vi "test caller.vi"() -> ()   [LabVIEW 2020]
uses:
  <userlib>/_NEVSTOP/Communicable State Machine(CSM)/Communicable State Machine.lvlib
  <userlib>/_NEVSTOP/Communicable State Machine(CSM)/_csmHelper/CSM-Helper.lvclass
  <userlib>/_NEVSTOP/Communicable State Machine(CSM)/_csmHelper/API/Destroy.vi
  <userlib>/_NEVSTOP/Communicable State Machine(CSM)/_csmHelper/API/Create From VI Reference.vi
  <userlib>/_NEVSTOP/Communicable State Machine(CSM)/_csmHelper/Properties/Read Back Tunnels Refs.vi
  <userlib>/_NEVSTOP/Communicable State Machine(CSM)/_Polymophic/Build No-Reply Asynchronous Message with Arguments.vi
panel:
  out "Array":string[](array[string])
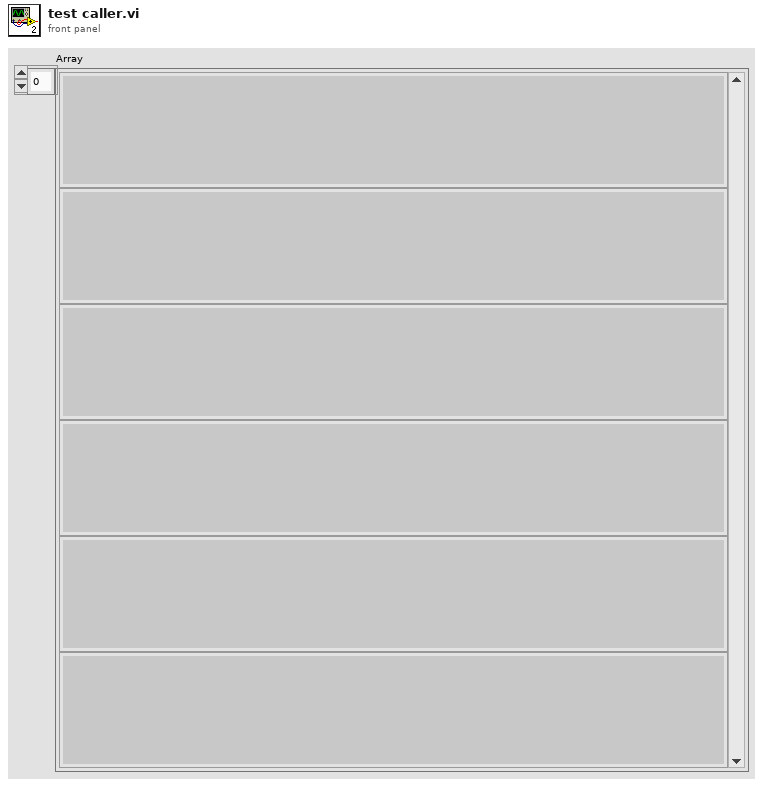
[diagram p1: front panel]
types:
  T1 = enum32{"Invalid", "Standard", "Closed", "Hidden", "Minimized", "Maximized"}
  T2 = enum32{"invalid app kind", "Development System", "Run Time System", "Student Edition", "Embedded LabVIEW", "Evaluation", "Custom"}
  T3 = typedef "Communicable State Machine.lvlib/_CSM_Response Source Message.ctl" = cluster{"‘State":string, "’Arguments":string, "’Error":errorcluster}
  T4 = cluster{"Core":cluster{"Current VI Reference":refnum<vi>, "Close Panel on Exit?":bool}, "Your Boolean data":bool, "Your string data":string}
  T5 = cluster{"Current VI Reference":refnum<vi>, "Close Panel on Exit?":bool}
  T6 = typedef "CSM-Helper.lvclass/_csmhelper_Back_Tunnels_Refs.ctl" = cluster{"Registration":refnum<vi>, "InternalData":refnum<vi>, "Resp":refnum<vi>, "Remaining State":refnum<vi>, "Error":refnum<vi>}
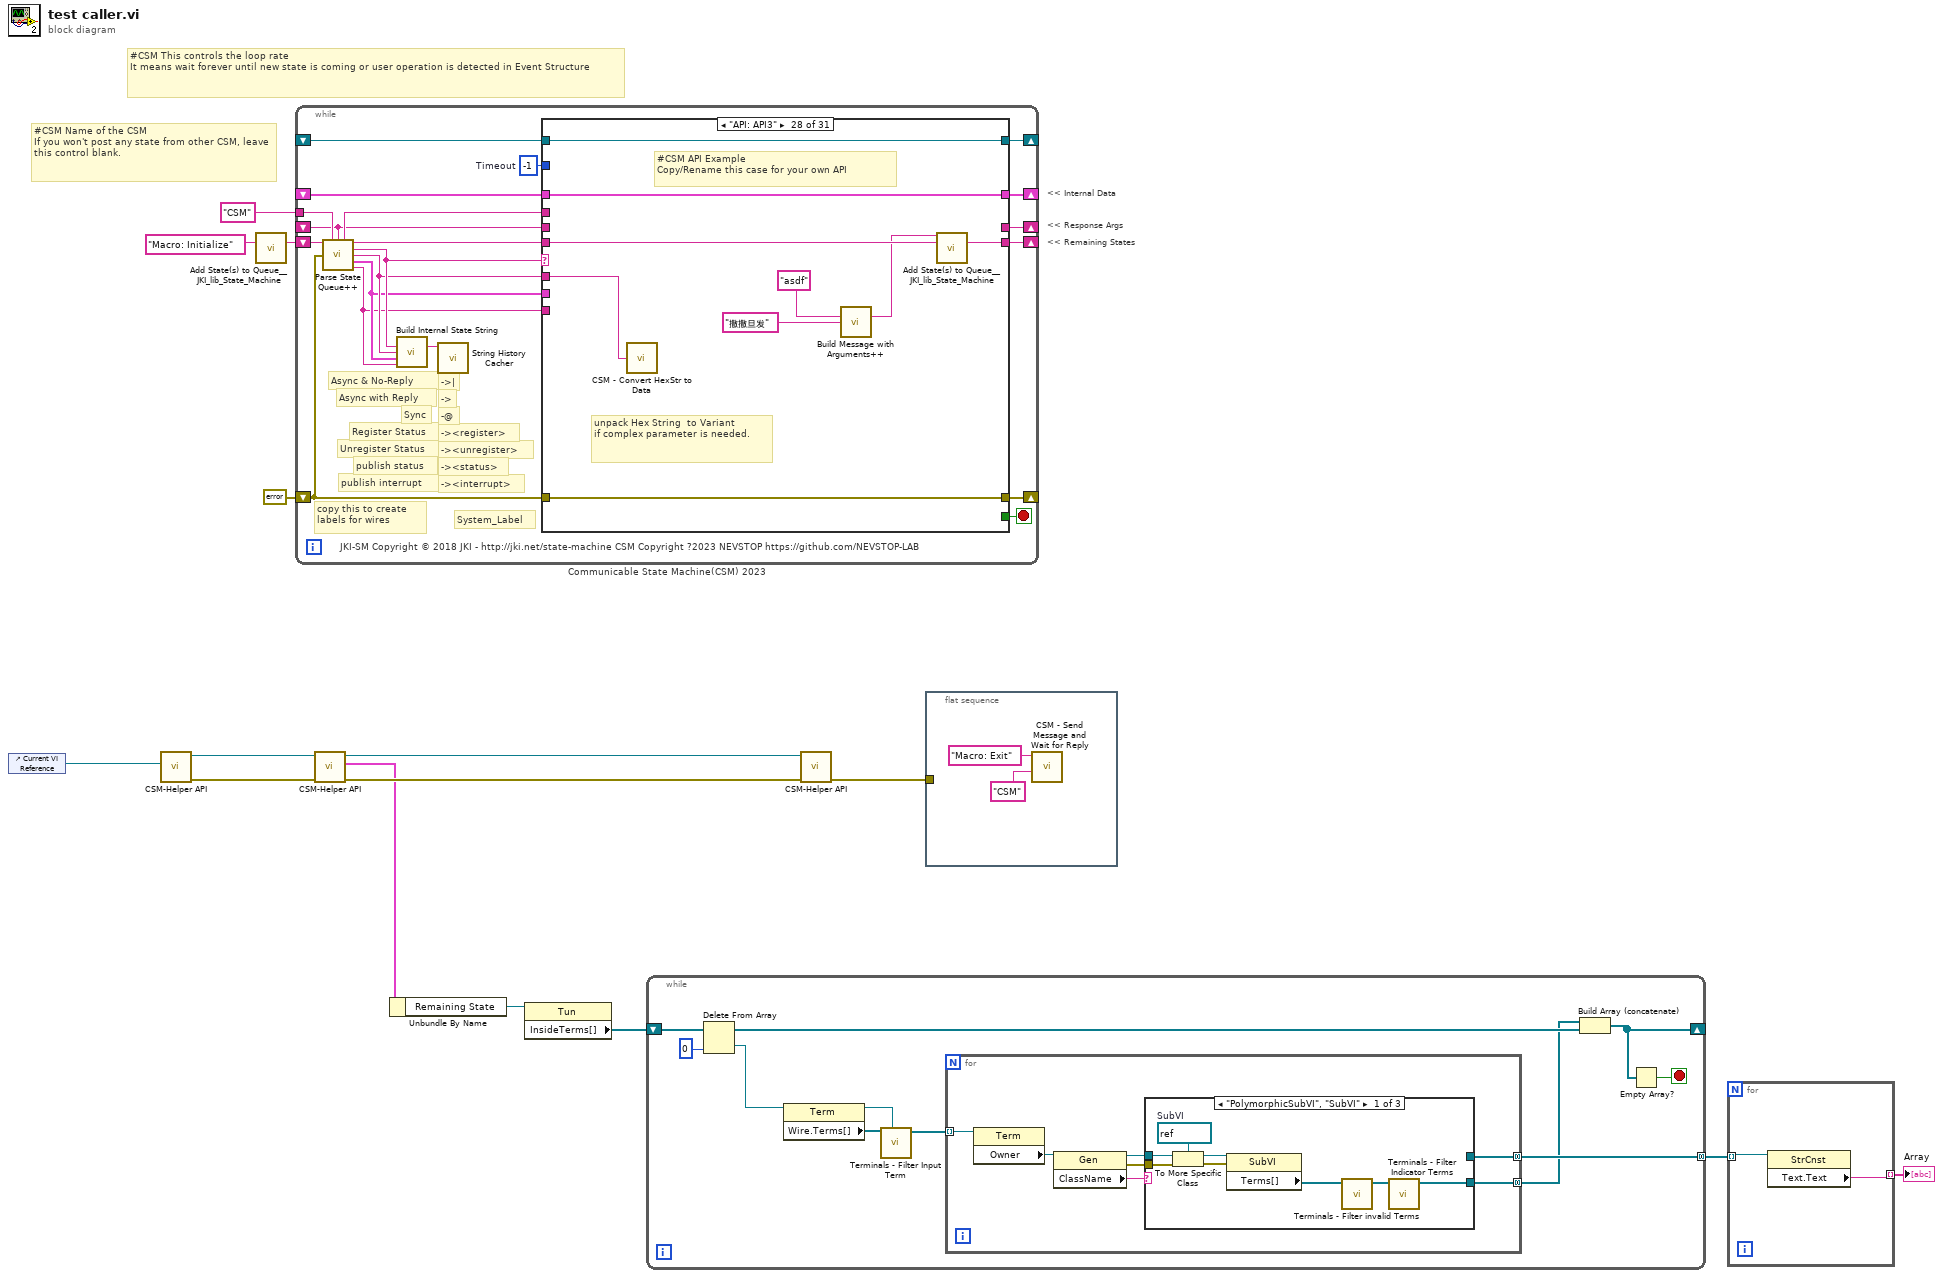
[diagram p0: block diagram]
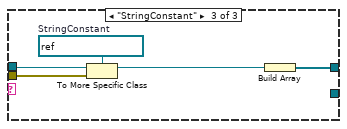
[diagram p3: hidden frame]
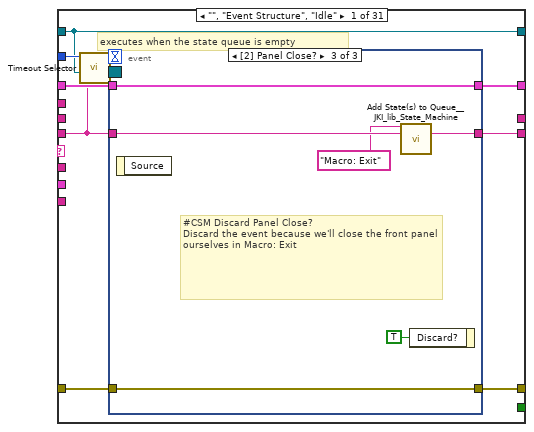
[diagram p4: hidden frame]
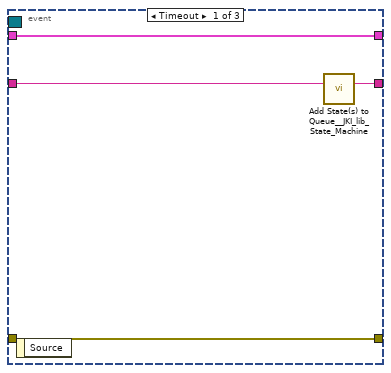
[diagram p5: hidden frame]
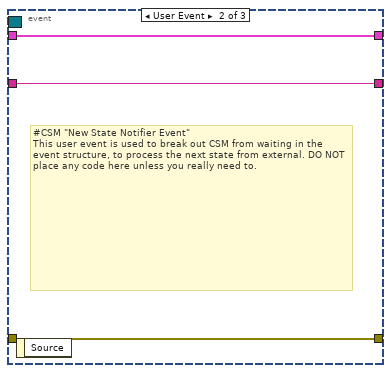
[diagram p6: hidden frame]
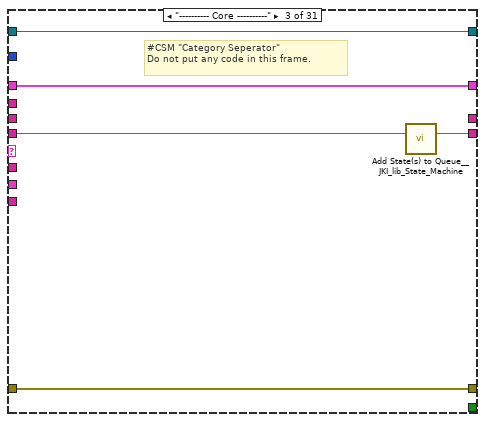
[diagram p8: hidden frame]
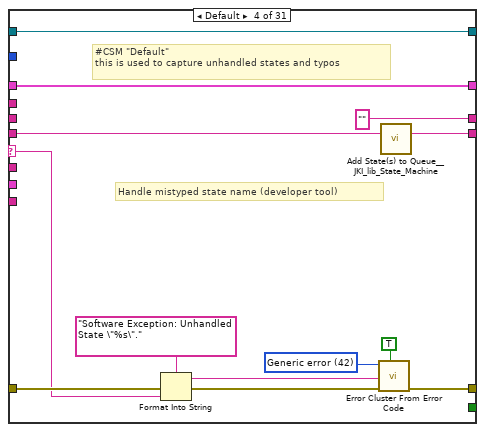
[diagram p9: hidden frame]
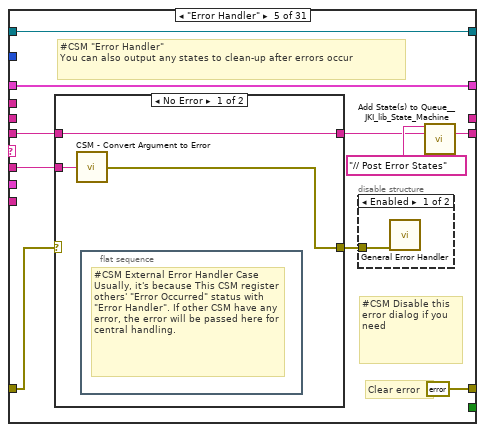
[diagram p10: hidden frame]
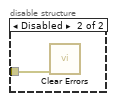
[diagram p11: hidden frame]
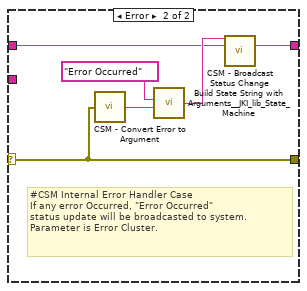
[diagram p12: hidden frame]
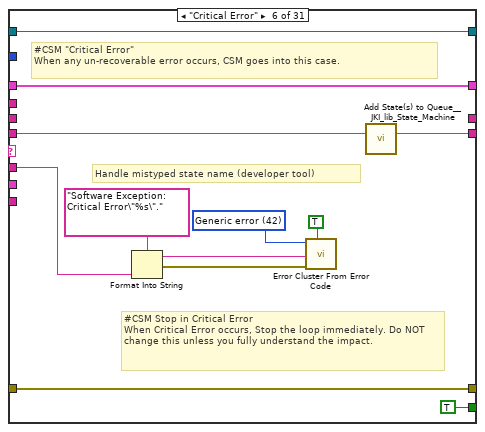
[diagram p13: hidden frame]
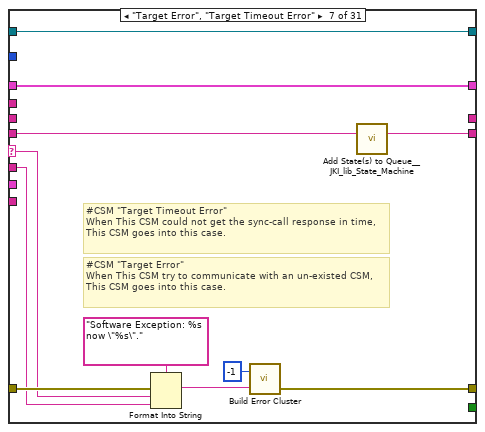
[diagram p14: hidden frame]
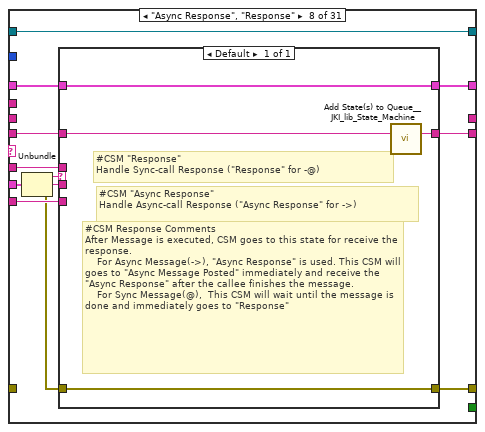
[diagram p15: hidden frame]
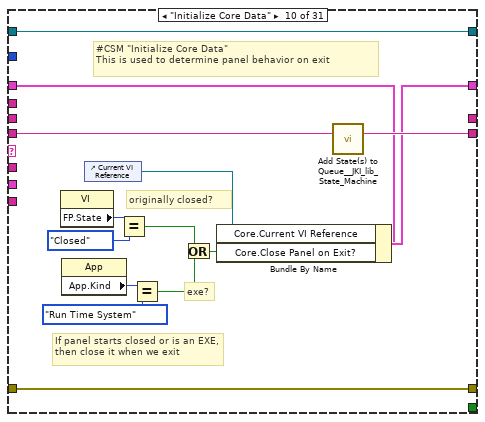
[diagram p17: hidden frame]
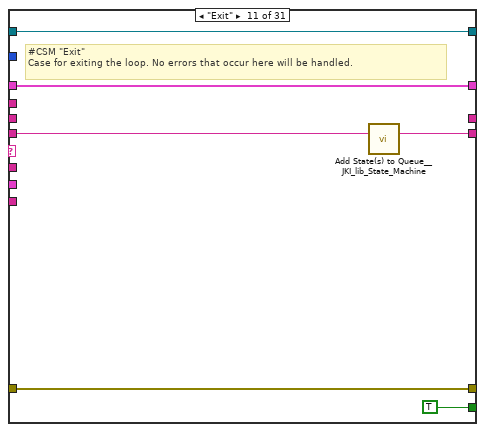
[diagram p18: hidden frame]
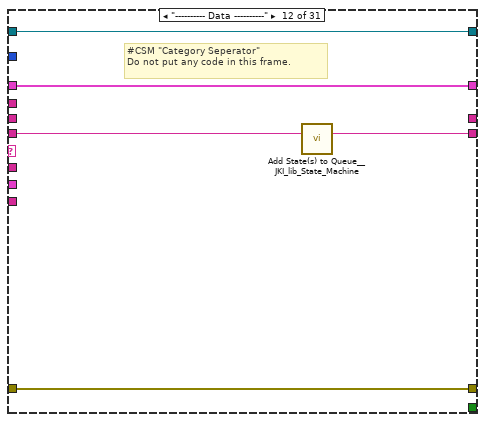
[diagram p19: hidden frame]
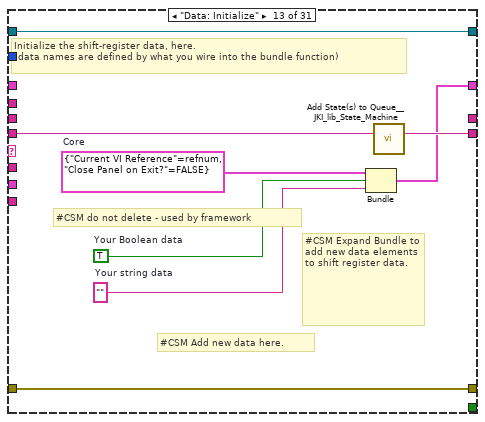
[diagram p20: hidden frame]
diagram:
  # "#CSM Name of the CSM\nIf you won't post any state from other CSM, leave this control blank."
  # "#CSM This controls the loop rate\nIt means wait forever until new state is coming or user operation is detected in Event Structure"
  # "<< Internal Data"
  # "<< Response Args"
  # "<< Remaining States"
  n1 = control-ref of="Current VI Reference"() -> (w15:refnum<vi>)
  n2 = call-poly <userlib>:"CSM-Helper API.vi"("VI"=w15) -> ("error out"=w9:errorcluster, "CSM-Helper.lvclass"=w8:refnum<class "CSM-Helper.lvclass">)  [unwired: 9 in]
  n3 = call <vilib>:"Add State(s) to Queue__JKI_lib_State_Machine.vi"("State(s) in (\"\")"="Macro: Initialize" ("Init State(\"Macro: Initialize\")")) -> ("States Out"=w10:string)  [unwired: 14 in]
  n4 = while "Communicable State Machine(CSM) 2023" {
    shift-right: [w30] -> _
    shift-left: _ -> [w29]
    shift-right: [w33] -> _
    shift-left: errorcluster {"status"=FALSE, "code"=0, "source"=""} ("error out") -> [w27]
    shift-right: [w32] -> _
    shift-left: w10 -> [w34]
    tunnel: "CSM" ("Name(\"\" to use uuid)") -> [w23]
    shift-right: [w26] -> _
    shift-left: _ -> [w16]
    shift-right: [w25] -> _
    shift-left: _ -> [w24]
    stop <- w31 stop-if-true
    w28 = -1  # Timeout
    # "-><interrupt>"
    # "-><status>"
    # "-><unregister>"
    # "-><register>"
    # "-@"
    # "->"
    # "->|"
    # "publish interrupt"
    # "publish status"
    # "Unregister Status"
    # "Register Status"
    # "Sync"
    # "Async with Reply"
    # "Async & No-Reply"
    # "copy this to create labels for wires"
    # "System_Label"
    # "JKI-SM Copyright © 2018 JKI - http://jki.net/state-machine CSM Copyright ?2023 NEVSTOP https://github.com/NEVSTOP-LAB"
    n5 = call <userlib>:"Parse State Queue++.vi"("State Queue"=w34, "Name(\"\" to use uuid)"=w23, "Response Arguments"=w16, "Error In (no error)"=w27) -> ("Name Used"=w17:string, "Remaining States"=w35:string, "Current State"=w21:string, "Arguments"=w20:string, ">> Response Source Message >>"=w19:T3, ">> Source CSM >>"=w18:string)  [unwired: 6 in]
    n6 = call <userlib>:"Build Internal State String.vi"("State"=w21, "Arguments (\"\")"=w20, ">> Response Source Message >>"=w19, "Source (\"\")"=w18) -> ("State with Arguments"=w22:string)  [unwired: 11 in]
    n7 = call <userlib>:"String History Cacher.vi"("String"=w22) -> ()  [unwired: 10 in, 1 out]
    n8 = case shown="\"API: API3\"" w21 {
      selector: w21 -> [_ _ _ w69 _ _ w116 _ _ _ _ _ _ _ _ _ _ _ _ _ _ _ _ _ _ _ _ _ _ _ _]
      tunnel: w35 -> [w36 w60 w66 w73 w84 w110 w118 w129 w142 w157 w163 w168 w176 w183 w188 w195 w199 w205 w210 w217 w233 w303 w311 w323 w326 w331 w337 w344 w354 w359 w364]
      tunnel: w20 -> [_ _ _ _ w83 w103 w117 w128 _ _ _ _ _ _ _ _ _ _ _ w212 w227 _ _ _ _ _ w334 w346 _ _ _]
      tunnel: w29 -> [w43 w59 w63 w71 w88 w111 w120 w131 w141 w150 w161 w165 _ w178 w185 w194 w198 w202 w208 w215 w229 w300 w308 w320 w325 w330 w336 w348 w351 w356 w361]
      tunnel: [w42 w61 w64 w75 errorcluster {"status"=FALSE, "code"=0, "source"=""} ("error out") w112 w114 w134 w143 w154 w160 w166 w173 w179 w186 w189 w197 w203 w207 w213 w230 w301 w309 w321 w327 w332 w338 w349 w352 w357 w362] -> w33
      tunnel: w27 -> [w41 w61 w64 w74 w85 w112 w122 _ w143 w154 w160 w166 w173 w180 w186 _ w200 w203 w207 w214 w231 w301 w309 w321 w327 w332 w338 w349 w352 w357 w362]
      tunnel: [w44 w60 w65 w72 w80 w109 w121 w130 w142 w156 w162 w167 w175 w182 w187 w195 w199 w204 w209 w216 w232 w302 w310 w322 w326 w331 w337 w345 w353 w358 w363] -> w32
      tunnel: [_ _ _ _ _ TRUE _ _ _ _ TRUE _ _ _ _ _ _ _ _ _ _ _ _ _ _ _ _ _ _ _ _] -> w31
      tunnel: [w40 w59 w63 w71 w88 w111 w120 w132 w141 w155 w161 w165 w174 w178 w185 w194 w198 w202 w208 w215 w229 w300 w308 w320 w325 w330 w336 w348 w351 w356 w361] -> w30
      tunnel: w28 -> [w39 _ _ _ _ _ _ _ _ _ _ _ _ _ _ _ _ _ _ _ _ _ _ _ _ _ _ _ _ _ _]
      tunnel: w18 -> [_ _ _ _ _ _ _ w126 _ _ _ _ _ _ _ _ _ _ _ _ _ _ _ _ _ _ _ _ _ _ _]
      tunnel: w19 -> [_ _ _ _ _ _ _ w133 _ _ _ _ _ _ _ _ _ _ _ _ _ _ _ _ _ _ _ _ _ _ _]
      tunnel: [_ _ _ "" _ _ _ _ _ _ _ _ _ _ _ _ _ _ _ _ _ _ _ _ _ "API1 Response" w333 _ _ _ _] -> w26
      tunnel: [w38 w58 w62 w67 w87 w101 w119 w135 w140 w144 w158 w164 w169 w177 w184 w193 w196 w201 w206 w211 w226 w299 w306 w314 w324 w329 w335 w347 w350 w355 w360] -> w25
      tunnel: w24 -> [w38 w58 w62 w67 w87 w101 w119 w135 w140 w144 w158 w164 w169 w177 w184 _ w196 w201 w206 w211 w226 w299 w306 w314 w324 w329 w335 w347 w350 w355 w360]
      tunnel: w17 -> [_ _ _ _ _ _ _ _ _ _ _ _ _ _ _ w192 _ _ _ _ _ _ _ _ _ _ _ _ _ _ _]
      tunnel: w16 -> [_ _ _ _ _ _ _ _ _ _ _ _ _ _ _ _ _ _ _ _ _ _ _ _ _ _ _ _ _ _ _]
      frame "", "Event Structure", "Idle" {
        # "executes when the state queue is empty"
        n9 = call <userlib>:"Timeout Selector.vi"("Remaining States"=w36, "Timeout Expected"=w39) -> ("Timeout"=w37:i32)  [unwired: 5 in]
        n10 = event shown="[2] Panel Close?" {
          selector: w38 -> [_ _ _]
          dyn-events: _ -> [_ _ _]
          timeout: w37 -> [_ _ _]
          tunnel: w36 -> [w48 w50 w57]
          tunnel: [w47 w50 w56] -> w44
          tunnel: w43 -> [w45 w51 w54]
          tunnel: [w46 w49 w55] -> w42
          tunnel: w41 -> [w46 w49 w55]
          tunnel: [w45 w51 w54] -> w40
          event Timeout {
            n11 = event-data() -> ()  [unwired: 1 in, 1 out]
            n12 = call <vilib>:"Add State(s) to Queue__JKI_lib_State_Machine.vi"("State(s) in (\"\")"=w48) -> ("States Out"=w47:string)  [unwired: 14 in]
          }
          event User Event {
            # "#CSM \"New State Notifier Event\"\nThis user event is used to break out CSM from waiting in the event structure, to process the next state from external. DO NOT place any code here unless you really need to."
            n13 = event-data() -> ()  [unwired: 1 in, 1 out]
          }
          event Panel Close? {
            # "#CSM Discard Panel Close?\nDiscard the event because we'll close the front panel ourselves in Macro: Exit"
            n14 = event-data() -> ()  [unwired: 1 in, 1 out]
            n15 = call <vilib>:"Add State(s) to Queue__JKI_lib_State_Machine.vi"("State(s) in Front (\"\")"="Macro: Exit", "State(s) in (\"\")"=w57) -> ("States Out"=w56:string)  [unwired: 13 in]
            n16 = event-data("Discard?"=TRUE) -> ()  [unwired: 1 in, 1 out]
          }
        }
      }
      frame "CSM Documentation" {
        # "#CSM README FIRST\n\nCommunicable State Machine(CSM) is a LabVIEW application framework that builds upon JKI State Machine(JKISM). It follows the pattern of JKISM and extends the keywords to describe message communication between modules, including concepts such as Sync-Message, Async-Message, Subscription/Unsubscription of status - essential elements for creating reusable code modules. For more information, please visit the CSM wiki: https://nevstop-lab.github.io/CSM-Wiki/\n\nFor instructions on JKI State Machine, visit: http://jki.net/state-machine/\nFor information about CSM, visit: https://github.com/NEVSTOP-LAB"
        # "#CSM \"Documentation\"\nCase for holding CSM Documenation"
      }
      frame "---------- Core ----------" {
        # "#CSM \"Category Seperator\"\nDo not put any code in this frame."
        n17 = call <vilib>:"Add State(s) to Queue__JKI_lib_State_Machine.vi"("State(s) in (\"\")"=w66) -> ("States Out"=w65:string)  [unwired: 14 in]
      }
      frame Default {
        w78 = 42 items=["No error", "Argument error", "Memory is full", "Out of zone", "End of file", "File already open", "Generic file I/O error", "File not found", "File permission error", "Disk is full", "Duplicate path", "Too many files open", "System feature not enabled", "Resource file not found", "Cannot add resource", "Resource not found", "Image not found", "Image memory error", "Pen does not exist", "Config type invalid", "Config token not found", "Config parse error", "Config memory error", "Bad external code format", "Bad external code offset", "External code not present", "Null window", "Destroy window error", "Null menu", "Print aborted", "Bad print record", "Print driver error", "Windows error during printing", "Memory error during printing", "Print dialog error", "Generic print error", "Invalid device refnum", "Device not found", "Device parameter error", "Device unit error", "Cannot open device", "Device call aborted", "Generic error", "Cancelled by user", "Object ID too low", "Object ID too high", "Object not in heap", "Unknown heap", "Unknown object (invalid DefProc)", "Unknown object (DefProc not in table)", "Message out of range", "Invalid (null) method", "Unknown message", "Manager call not supported", "Bad address", "Network operation in progress", "Network operation timed out", "Connection is busy", "Network attribute not supported", "Network error", "Address in use", "System out of memory", "Connection aborted", "Connection refused", "Not connected", "Already connected", "Connection closed", "Initialization error (interapplication manager)", "Bad occurrence", "Wait on unbound occurrence handler", "Occurrence queue overflow", "Datalog type conflict", "Unused", "Unrecognized type (interapplication manager)", "Memory corrupt", "Failed to make temporary DLL", "Old CIN version", "Drag socket not found", "Failed to load drop-object", "Failed to register OLE object", "Failed to release OLE object", "Format specifier type mismatch", "Unknown format specifier", "Too few format specifiers", "Too many format specifiers", "Scan failed", "Newer CIN version", "Error converting to variant", "Runtime menu error", "Password tampered", "Variant attribute not found", "Incompatible variant data type", "Event data is not available", "Event Store is not present", "Occurrence is not found", "Event Queue is not created", "Event info is not available", "Refnum passed is NULL", "Error retrieving Class GUID", "Error retrieving CoClass GUID", "Error retrieving TypeLib GUID.", "Bad built application magic bytes.", "Specific driver is different from the specific driver associated with the Logical Name.", "There is no session opened to the class driver.", "Max Error", "MAX - Error with config objects", "MAX - Error loading configuration", "MAX - Group not supported"]
        # "#CSM \"Default\"\nthis is used to capture unhandled states and typos"
        # "Handle mistyped state name (developer tool)"
        n18 = Format Into String(format string="Software Exception: Unhandled State \"%s\"." ("message"), error in=w74, w69) -> (resulting string=w77:string, error out=w76:errorcluster)  [unwired: 1 in]
        n19 = call <vilib>:"Error Cluster From Error Code.vi"("show call chain? (False)"=TRUE, "error in (no error)"=w76, "error message (\"\")"=w77, "error code (0)"=w78) -> ("error out"=w75:errorcluster)  [unwired: 5 in]
        n20 = call <vilib>:"Add State(s) to Queue__JKI_lib_State_Machine.vi"("State(s) in (\"\")"=w73) -> ("States Out"=w72:string)  [unwired: 14 in]
      }
      frame "Error Handler" {
        # "#CSM Disable this error dialog if you need"
        # "#CSM \"Error Handler\"\nYou can also output any states to clean-up after errors occur"
        # "Clear error"
        n21 = case shown="No Error" w85 {
          selector: w85 -> [_ w95]
          tunnel: [w94 w97] -> w81
          tunnel: w84 -> [w94 w96]
          tunnel: w83 -> [w93 _]
          tunnel: [w92 w95] -> w86
          frame No Error {
            n22 = call <userlib>:"CSM - Convert Argument to Error.vi"("Argument"=w93) -> ("error"=w92:errorcluster)  [unwired: 4 in]
            n23 = flat-sequence {
              frame #0 {
                # "#CSM External Error Handler Case\nUsually, it's because This CSM register others' \"Error Occurred\" status with \"Error Handler\". If other CSM have any error, the error will be passed here for central handling."
              }
            }
          }
          frame Error {
            # "#CSM Internal Error Handler Case \nIf any error Occurred, \"Error Occurred\" \nstatus update will be broadcasted to system.\nParameter is Error Cluster."
            n24 = call <userlib>:"CSM - Convert Error to Argument.vi"("error in (no error)"=w95) -> ("Arguments"=w99:string)  [unwired: 4 in]
            n25 = call <vilib>:"Build State String with Arguments__JKI_lib_State_Machine.vi"("Arguments (\"\")"=w99, "State"="Error Occurred" ("Status with Arguments")) -> ("State with Arguments"=w98:string)  [unwired: 4 in]
            n26 = call <userlib>:"CSM - Broadcast Status Change.vi"("Status with Arguments"=w98, "State Queue"=w96) -> ("Remaining States"=w97:string)  [unwired: 13 in]
          }
        }
        n27 = disable-structure shown="Enabled" {
          disable-tunnel: w86 -> [w90 w91]
          frame Enabled {
            n28 = call <vilib>:"General Error Handler.vi"("error in (no error)"=w90) -> ()  [unwired: 10 in, 5 out]
          }
          frame Disabled {
            n29 = call <vilib>:"Clear Errors.vi"("error in (no error)"=w91) -> ()  [unwired: 5 in, 2 out]
          }
        }
        n30 = call <vilib>:"Add State(s) to Queue__JKI_lib_State_Machine.vi"("State(s) in Front (\"\")"="// Post Error States", "State(s) in (\"\")"=w81) -> ("States Out"=w80:string)  [unwired: 13 in]
      }
      frame "Critical Error" {
        w107 = 42 items=["No error", "Argument error", "Memory is full", "Out of zone", "End of file", "File already open", "Generic file I/O error", "File not found", "File permission error", "Disk is full", "Duplicate path", "Too many files open", "System feature not enabled", "Resource file not found", "Cannot add resource", "Resource not found", "Image not found", "Image memory error", "Pen does not exist", "Config type invalid", "Config token not found", "Config parse error", "Config memory error", "Bad external code format", "Bad external code offset", "External code not present", "Null window", "Destroy window error", "Null menu", "Print aborted", "Bad print record", "Print driver error", "Windows error during printing", "Memory error during printing", "Print dialog error", "Generic print error", "Invalid device refnum", "Device not found", "Device parameter error", "Device unit error", "Cannot open device", "Device call aborted", "Generic error", "Cancelled by user", "Object ID too low", "Object ID too high", "Object not in heap", "Unknown heap", "Unknown object (invalid DefProc)", "Unknown object (DefProc not in table)", "Message out of range", "Invalid (null) method", "Unknown message", "Manager call not supported", "Bad address", "Network operation in progress", "Network operation timed out", "Connection is busy", "Network attribute not supported", "Network error", "Address in use", "System out of memory", "Connection aborted", "Connection refused", "Not connected", "Already connected", "Connection closed", "Initialization error (interapplication manager)", "Bad occurrence", "Wait on unbound occurrence handler", "Occurrence queue overflow", "Datalog type conflict", "Unused", "Unrecognized type (interapplication manager)", "Memory corrupt", "Failed to make temporary DLL", "Old CIN version", "Drag socket not found", "Failed to load drop-object", "Failed to register OLE object", "Failed to release OLE object", "Format specifier type mismatch", "Unknown format specifier", "Too few format specifiers", "Too many format specifiers", "Scan failed", "Newer CIN version", "Error converting to variant", "Runtime menu error", "Password tampered", "Variant attribute not found", "Incompatible variant data type", "Event data is not available", "Event Store is not present", "Occurrence is not found", "Event Queue is not created", "Event info is not available", "Refnum passed is NULL", "Error retrieving Class GUID", "Error retrieving CoClass GUID", "Error retrieving TypeLib GUID.", "Bad built application magic bytes.", "Specific driver is different from the specific driver associated with the Logical Name.", "There is no session opened to the class driver.", "Max Error", "MAX - Error with config objects", "MAX - Error loading configuration", "MAX - Group not supported"]
        # "#CSM Stop in Critical Error\nWhen Critical Error occurs, Stop the loop immediately. Do NOT change this unless you fully understand the impact."
        # "#CSM \"Critical Error\"\nWhen any un-recoverable error occurs, CSM goes into this case."
        # "Handle mistyped state name (developer tool)"
        n31 = Format Into String(format string="Software Exception: Critical Error\"%s\"." ("message"), w103) -> (resulting string=w106:string, error out=w105:errorcluster)  [unwired: 2 in]
        n32 = call <vilib>:"Error Cluster From Error Code.vi"("show call chain? (False)"=TRUE, "error in (no error)"=w105, "error message (\"\")"=w106, "error code (0)"=w107) -> ()  [unwired: 5 in, 1 out]
        n33 = call <vilib>:"Add State(s) to Queue__JKI_lib_State_Machine.vi"("State(s) in (\"\")"=w110) -> ("States Out"=w109:string)  [unwired: 14 in]
      }
      frame "Target Error", "Target Timeout Error" {
        # "#CSM \"Target Error\"\nWhen This CSM try to communicate with an un-existed CSM, This CSM goes into this case."
        # "#CSM \"Target Timeout Error\"\nWhen This CSM could not get the sync-call response in time, This CSM goes into this case."
        n34 = Format Into String(format string="Software Exception: %s now \"%s\"." ("message"), error in=w122, w116, w117) -> (resulting string=w115:string)  [unwired: 1 in, 1 out]
        n35 = call <userlib>:"Build Error Cluster.vi"("String to Prepend to source (\"\")"=w115, "code"=-1) -> ("error out"=w114:errorcluster)
        n36 = call <vilib>:"Add State(s) to Queue__JKI_lib_State_Machine.vi"("State(s) in (\"\")"=w118) -> ("States Out"=w121:string)  [unwired: 14 in]
      }
      frame "Async Response", "Response" {
        n37 = Unbundle(w133) -> ("‘State"=w127:string, "’Arguments"=w125:string, "’Error"=w124:errorcluster)
        n38 = case shown="Default" w127 {
          tunnel: [w139] -> w134
          tunnel: w124 -> [w139]
          tunnel: [w138] -> w132
          tunnel: w131 -> [w138]
          tunnel: [w136] -> w130
          tunnel: w129 -> [w137]
          tunnel: w128 -> [_]
          tunnel: w126 -> [_]
          tunnel: w125 -> [_]
          frame Default {
            # "#CSM Response Comments\nAfter Message is executed, CSM goes to this state for receive the response.\n    For Async Message(->), \"Async Response\" is used. This CSM will goes to \"Async Message Posted\" immediately and receive the \"Async Response\" after the callee finishes the message.\n    For Sync Message(@),  This CSM will wait until the message is done and immediately goes to \"Response\""
            # "#CSM \"Async Response\"\nHandle Async-call Response (\"Async Response\" for ->)"
            # "#CSM \"Response\"\nHandle Sync-call Response (\"Response\" for -@)"
            n39 = call <vilib>:"Add State(s) to Queue__JKI_lib_State_Machine.vi"("State(s) in (\"\")"=w137) -> ("States Out"=w136:string)  [unwired: 14 in]
          }
        }
      }
      frame "Async Message Posted" {
        # "#CSM \"Async Message Posted\"\nAfter Async Message is posted (-> or ->| ), CSM goes to this state for post-action.\nYou can use Argument - State to tell which Async Message is called."
      }
      frame "Initialize Core Data" {
        # "#CSM \"Initialize Core Data\"\nThis is used to determine panel behavior on exit"
        # "originally closed?"
        # "exe?"
        # "If panel starts closed or is an EXE, then close it when we exit"
        n40 = property class="VI"() -> ("FP.State"=w147:T1)  [unwired: 2 in, 2 out]
        n41 = property class="App"() -> ("App.Kind"=w153:T2)  [unwired: 2 in, 2 out]
        n42 = control-ref of="Current VI Reference"() -> (w148:refnum<vi>)
        n43 = Equal?(x=w147, y=T1."Closed" ("Front Panel Window:State")) -> (x = y?=w145:bool)
        n44 = Equal?(x=w153, y=T2."Run Time System" ("Application:Kind")) -> (x = y?=w151:bool)
        n45 = Or(x=w145, y=w151) -> (x .or. y?=w149:bool)
        n46 = Bundle By Name(cluster=w150, "Core.Current VI Reference"=w148, "Core.Close Panel on Exit?"=w149) -> (w155:T4)
        n47 = call <vilib>:"Add State(s) to Queue__JKI_lib_State_Machine.vi"("State(s) in (\"\")"=w157) -> ("States Out"=w156:string)  [unwired: 14 in]
      }
      frame "Exit" {
        # "#CSM \"Exit\"\nCase for exiting the loop. No errors that occur here will be handled."
        n48 = call <vilib>:"Add State(s) to Queue__JKI_lib_State_Machine.vi"("State(s) in (\"\")"=w163) -> ("States Out"=w162:string)  [unwired: 14 in]
      }
      frame "---------- Data ----------" {
        # "#CSM \"Category Seperator\"\nDo not put any code in this frame."
        n49 = call <vilib>:"Add State(s) to Queue__JKI_lib_State_Machine.vi"("State(s) in (\"\")"=w168) -> ("States Out"=w167:string)  [unwired: 14 in]
      }
      frame "Data: Initialize" {
        w170 = T5 {"Current VI Reference"=refnum, "Close Panel on Exit?"=FALSE}  # Core
        w172 = TRUE  # Your Boolean data
        w171 = ""  # Your string data
        # "#CSM do not delete - used by framework"
        # "#CSM Expand Bundle to add new data elements to shift register data."
        # "#CSM Add new data here."
        # "Initialize the shift-register data, here.\n(data names are defined by what you wire into the bundle function)"
        n50 = Bundle("Core"=w170, "Your Boolean data"=w172, "Your string data"=w171) -> (w174:T4)  [unwired: 1 in]
        n51 = call <vilib>:"Add State(s) to Queue__JKI_lib_State_Machine.vi"("State(s) in (\"\")"=w176) -> ("States Out"=w175:string)  [unwired: 14 in]
      }
      frame "Data: Cleanup" {
        # "Cleanup any data and references, here.\n(this is called automatically, by the Macro: Exit)"
        n52 = Unbundle By Name(w178) -> ("Core.Current VI Reference"=w181:refnum<vi>)
        n53 = Close Reference(reference=w181, error in (no error)=w180) -> (error out=w179:errorcluster)
        n54 = call <vilib>:"Add State(s) to Queue__JKI_lib_State_Machine.vi"("State(s) in (\"\")"=w183) -> ("States Out"=w182:string)  [unwired: 14 in]
      }
      frame "---------- Events ----------" {
        # "#CSM \"Category Seperator\"\nDo not put any code in this frame."
        n55 = call <vilib>:"Add State(s) to Queue__JKI_lib_State_Machine.vi"("State(s) in (\"\")"=w188) -> ("States Out"=w187:string)  [unwired: 14 in]
      }
      frame "Events: Register" {
        # "#CSM \"Events: Register\"\nRegister user event. New Message Event is registered to break CSM waiting in event structure by default."
        # "#CSM Register New Message Event\nRegister message event to break Waiting in Event structure."
        n56 = call <userlib>:"CSM - Get New State Notifier Event.vi"("Name(\"\" to use uuid) in"=w192) -> ("Error out"=w190:errorcluster, "New State Notifier Event"=w191:refnum<user-event>)  [unwired: 9 in]
        n57 = register-events(error in=w190, w191) -> (reference out=w193:refnum<event-registration>, error out=w189:errorcluster)  [unwired: 1 in]
      }
      frame "Events: Unregister" {
        # "#CSM \"Events: Unregister\"\nUnregister user event."
        n58 = Unregister For Events(event registration refnum=w196, error in=w200) -> (error out=w197:errorcluster)
      }
      frame "---------- UI ----------" {
        # "#CSM \"Category Seperator\"\nDo not put any code in this frame."
        n59 = call <vilib>:"Add State(s) to Queue__JKI_lib_State_Machine.vi"("State(s) in (\"\")"=w205) -> ("States Out"=w204:string)  [unwired: 14 in]
      }
      frame "UI: Initialize" {
        # "#CSM \"UI: Initialize\"\nInitialize the User Interface, here.\n(this is called automatically, by the Macro: Init)"
        n60 = call <vilib>:"Add State(s) to Queue__JKI_lib_State_Machine.vi"("State(s) in (\"\")"=w210) -> ("States Out"=w209:string)  [unwired: 14 in]
      }
      frame "UI: Cursor Set" {
        # "#CSM \"UI: Cursor Set\"\nSet and Unset Cursor Busy.\n(Usage: \"UI: Cursor Set >> Busy|Idle\")"
        # "Argument"
        n61 = disable-structure shown="TARGET_TYPE!=Windows" {
          disable-tunnel: w214 -> [w220 w225]
          disable-tunnel: [w219 w225] -> w213
          disable-tunnel: w212 -> [w218 _]
          frame condition #0 (active) {
            n62 = case shown="\"Idle\", Default" w218 {
              tunnel: w220 -> [w222 w224]
              tunnel: [w221 w223] -> w219
              frame "Idle", Default {
                n63 = call <vilib>:"Unset Busy.vi"("error in (no error)"=w222) -> ("error out"=w221:errorcluster)  [unwired: 10 in]
              }
              frame "Busy" {
                n64 = call <vilib>:"Set Busy.vi"("error in (no error)"=w224) -> ("error out"=w223:errorcluster)  [unwired: 9 in, 1 out]
              }
            }
          }
          frame condition #1 {
          }
        }
        n65 = call <vilib>:"Add State(s) to Queue__JKI_lib_State_Machine.vi"("State(s) in (\"\")"=w217) -> ("States Out"=w216:string)  [unwired: 14 in]
      }
      frame "UI: Front Panel State" {
        # "#CSM \"UI: Front Panel State\"\nSet Front Panel Open or Closed\n(Usage: \"UI: Front Panel State >> Open|Close\")"
        # "Argument"
        n66 = Unbundle By Name(w229) -> ("Core.Current VI Reference"=w228:refnum<vi>)
        n67 = call <vilib>:"Add State(s) to Queue__JKI_lib_State_Machine.vi"("State(s) in (\"\")"=w233) -> ("States Out"=w232:string)  [unwired: 14 in]
        n68 = case shown="\"Close\", \"Closed\"" w227 {
          tunnel: w231 -> [w239 w254 w265 w278 w291]
          tunnel: [w241 w255 w267 w280 w293] -> w230
          tunnel: w228 -> [w240 w252 w266 w279 w292]
          frame "Open", "Standard", Default {
            w234 = T1."Standard" ("State")
            n69 = property class="VI"(reference=w240, error in=w239) -> (reference out=w237:refnum<vi>, error out=w238:errorcluster, "FP.State"=w236:T1)
            n70 = Not Equal?(x=w236, y=w234) -> (x != y?=w235:bool)
            n71 = case shown="True" w235 {
              tunnel: [w245 w247] -> w241
              tunnel: w238 -> [w244 w247]
              tunnel: w237 -> [w243 _]
              tunnel: w234 -> [w242 _]
              frame True {
                n72 = invoke class="VI" method="FP.Open"(reference=w243, error in=w244, "Activate"=TRUE, "State"=w242) -> (error out=w245:errorcluster)  [unwired: 1 in, 4 out]
              }
              frame False {
              }
            }
          }
          frame "Close", "Closed" {
            n73 = property class="VI"(reference=w252, error in=w254) -> (reference out=w251:refnum<vi>, error out=w253:errorcluster, "FP.State"=w249:T1)
            n74 = Not Equal?(x=w249, y=T1."Closed" ("Front Panel Window:State")) -> (x != y?=w248:bool)
            n75 = case shown="False" w248 {
              tunnel: [w256 w259] -> w255
              tunnel: w253 -> [w256 w258]
              tunnel: w251 -> [_ w257]
              frame False {
              }
              frame True {
                n76 = invoke class="VI" method="FP.Close"(reference=w257, error in=w258) -> (error out=w259:errorcluster)  [unwired: 1 in, 2 out]
              }
            }
          }
          frame "Hidden", "Hide" {
            w260 = T1."Hidden" ("State")
            n77 = property class="VI"(reference=w266, error in=w265) -> (reference out=w263:refnum<vi>, error out=w264:errorcluster, "FP.State"=w262:T1)
            n78 = Not Equal?(x=w262, y=w260) -> (x != y?=w261:bool)
            n79 = case shown="True" w261 {
              tunnel: [w271 w272] -> w267
              tunnel: w264 -> [w270 w272]
              tunnel: w263 -> [w269 _]
              tunnel: w260 -> [w268 _]
              frame True {
                n80 = invoke class="VI" method="FP.Open"(reference=w269, error in=w270, "State"=w268) -> (error out=w271:errorcluster)  [unwired: 2 in, 4 out]
              }
              frame False {
              }
            }
          }
          frame "Minimize", "Minimized" {
            w273 = T1."Minimized" ("State")
            n81 = property class="VI"(reference=w279, error in=w278) -> (reference out=w276:refnum<vi>, error out=w277:errorcluster, "FP.State"=w275:T1)
            n82 = Not Equal?(x=w275, y=w273) -> (x != y?=w274:bool)
            n83 = case shown="True" w274 {
              tunnel: [w284 w285] -> w280
              tunnel: w277 -> [w283 w285]
              tunnel: w276 -> [w282 _]
              tunnel: w273 -> [w281 _]
              frame True {
                n84 = invoke class="VI" method="FP.Open"(reference=w282, error in=w283, "State"=w281) -> (error out=w284:errorcluster)  [unwired: 2 in, 4 out]
              }
              frame False {
              }
            }
          }
          frame "Maximize", "Maximized" {
            w286 = T1."Maximized" ("State")
            n85 = property class="VI"(reference=w292, error in=w291) -> (reference out=w289:refnum<vi>, error out=w290:errorcluster, "FP.State"=w288:T1)
            n86 = Not Equal?(x=w288, y=w286) -> (x != y?=w287:bool)
            n87 = case shown="True" w287 {
              tunnel: [w297 w298] -> w293
              tunnel: w290 -> [w296 w298]
              tunnel: w289 -> [w295 _]
              tunnel: w286 -> [w294 _]
              frame True {
                n88 = invoke class="VI" method="FP.Open"(reference=w295, error in=w296, "State"=w294) -> (error out=w297:errorcluster)  [unwired: 2 in, 4 out]
              }
              frame False {
              }
            }
          }
        }
      }
      frame "---------- Macro ----------" {
        # "#CSM \"Category Seperator\"\nDo not put any code in this frame."
        n89 = call <vilib>:"Add State(s) to Queue__JKI_lib_State_Machine.vi"("State(s) in (\"\")"=w303) -> ("States Out"=w302:string)  [unwired: 14 in]
      }
      frame "Macro: Initialize" {
        w305 = "Data: Initialize2\nInitialize Core Data\nEvents: Register\nUI: Initialize\nUI: Front Panel State >> Open"  # Data: Initialize2 Initialize Core Data Events: Register UI: Initialize UI: Front Panel State >> Open
        w307 = "Data: Initialize\nInitialize Core Data\nEvents: Register\nUI: Initialize\nUI: Front Panel State >> Open"  # Data: Initialize Initialize Core Data Events: Register UI: Initialize UI: Front Panel State >> Open
        # "#CSM \"Macro: Initialize\"\nInitialization Macro (This is called once, when the VI starts)"
        n90 = call <vilib>:"Add State(s) to Queue__JKI_lib_State_Machine.vi"("State(s) in (\"\")"=w305) -> ("States Out"=w304:string)  [unwired: 14 in]
        n91 = call <vilib>:"Add State(s) to Queue__JKI_lib_State_Machine.vi"("State(s) in Front (\"\")"=w307, "State(s) in (\"\")"=w311, "State(s) at Back (\"\")"=w304) -> ("States Out"=w310:string)  [unwired: 12 in]
      }
      frame "Macro: Exit" {
        # "#CSM \"Macro: Exit\"\nExit Macro (This is called once, when the VI exits)"
        n92 = Unbundle By Name(w320) -> ("Core.Close Panel on Exit?"=w319:bool)
        n93 = Select(t="UI: Front Panel State >> Close", s=w319, f="") -> (s? t:f=w316:string)
        n94 = call <vilib>:"Add State(s) to Queue__JKI_lib_State_Machine.vi"("State(s) in Front (\"\")"="//Exit Sub-Modules ", "State(s) in (\"\")"=w316, "State(s) at Back (\"\")"="Data: Cleanup\nEvents: Unregister\nExit") -> ("States Out"=w312:string)  [unwired: 12 in]
        n95 = call <vilib>:"Add State(s) to Queue__JKI_lib_State_Machine.vi"("State(s) in Front (\"\")"=w312, "State(s) in (\"\")"=w323) -> ("States Out"=w322:string)  [unwired: 13 in]
      }
      frame "---------- API ----------" {
        # "#CSM \"Category Seperator\"\nDo not put any code in this frame."
      }
      frame "API: API1" {
        # "#CSM API Example\nCopy/Rename this case for your own API"
        # "#CSM Response\nConnect this to return the response of your API"
        # "#CSM >> Source CSM >>\nIf you need to tell who triggered this state , use this string. If it's this case itself, this string is \"\"."
        # "#CSM >> Arguments >>\nDeal with the parameter if any"
      }
      frame "API: API2" {
        # "#CSM API Example\nCopy/Rename this case for your own API"
        # "unpack Hex String  to Variant\nif complex parameter is needed."
        n96 = call <userlib>:"CSM - Convert HexStr to Data.vi"("HEX String"=w334) -> ()  [unwired: 7 in, 2 out]
        n97 = disable-structure shown="Disabled" {
          disable-tunnel: [w339 "API2 Response"] -> w333
          frame Disabled {
            # "pack variant to hexstr \nif complex response is needed."
            # "complex Response"
            n98 = call <userlib>:"CSM - Convert Data to HexStr.vi"() -> ("HEX String (0-9,A-F)"=w339:string)  [unwired: 9 in]
          }
          frame Enabled {
          }
        }
      }
      frame "API: API3" {
        # "#CSM API Example\nCopy/Rename this case for your own API"
        # "unpack Hex String  to Variant\nif complex parameter is needed."
        n99 = call <userlib>:"CSM - Convert HexStr to Data.vi"("HEX String"=w346) -> ()  [unwired: 7 in, 2 out]
        n100 = call-poly <userlib>:"Build Message with Arguments++.vi"("State with Arguments"="asdf", "Arguments (\"\")"="撒撒旦发" ("Arguments (\"\")")) -> ("State with Arguments out"=w341:string)  [unwired: 13 in]
        n101 = call <vilib>:"Add State(s) to Queue__JKI_lib_State_Machine.vi"("State(s) in Front (\"\")"=w341, "State(s) in (\"\")"=w344) -> ("States Out"=w345:string)  [unwired: 13 in]
      }
      frame "---------- Action ----------" {
        # "#CSM \"Category Seperator\"\nDo not put any code in this frame."
        n102 = call <vilib>:"Add State(s) to Queue__JKI_lib_State_Machine.vi"("State(s) in (\"\")"=w354) -> ("States Out"=w353:string)  [unwired: 14 in]
      }
      frame "Action: action1" {
        # "#CSM \"Internal State\"\nThis category is used for holding internal states"
        n103 = call <vilib>:"Add State(s) to Queue__JKI_lib_State_Machine.vi"("State(s) in (\"\")"=w359) -> ("States Out"=w358:string)  [unwired: 14 in]
      }
      frame "Action: action2" {
        # "#CSM \"Internal State\"\nThis category is used for holding internal states"
        n104 = call <vilib>:"Add State(s) to Queue__JKI_lib_State_Machine.vi"("State(s) in (\"\")"=w364) -> ("States Out"=w363:string)  [unwired: 14 in]
      }
    }
  }
  n105 = call-poly <userlib>:"CSM-Helper API.vi"("error in (no error)"=w9, "CSM-Helper in"=w8) -> ("error out"=w6:errorcluster, "Back Tunnels"=w5:T6, "CSM-Helper out"=w7:refnum<class "CSM-Helper.lvclass">)  [unwired: 7 in]
  n106 = Unbundle By Name(w5) -> ("Remaining State"=w4:refnum<vi>)
  n107 = property class="Tun"(reference=w4) -> ("InsideTerms[]"=w3:refnum<vi>[])  [unwired: 1 in, 2 out]
  n108 = while {
    shift-right: [w367] -> _
    shift-left: w3 -> [w375]
    tunnel: [w370] -> w2 mode=concatenating
    stop <- w369 stop-if-true
    n109 = Delete From Array(array=w375, index=0) -> (deleted portion=w371:refnum<vi>, array with subset deleted=w368:refnum<vi>[])  [unwired: 1 in]
    n110 = property class="Term"(reference=w371) -> (reference out=w373:refnum<vi>, "Wire.Terms[]"=w374:refnum<vi>[])  [unwired: 1 in, 1 out]
    n111 = call <userlib>:"Terminals - Filter Input Term.vi"("InnerTerminal in"=w373, "Wire.Terms[] in"=w374) -> ("Wire.Terms[] out"=w365:refnum<vi>[])  [unwired: 9 in]
    n112 = for {
      tunnel: w365 -> [w382] mode=indexing
      tunnel: [w377] -> w370 mode=concatenating
      tunnel: [w376] -> w366 mode=concatenating
      n113 = property class="Term"(reference=w382) -> ("Owner"=w381:refnum<vi>)  [unwired: 1 in, 2 out]
      n114 = property class="Gen"(reference=w381) -> (reference out=w379:refnum<vi>, error out=w378:errorcluster, "ClassName"=w380:string)  [unwired: 1 in]
      n115 = case shown="\"PolymorphicSubVI\", \"SubVI\"" w380 {
        tunnel: w379 -> [w389 _ w395]
        tunnel: w378 -> [w388 _ w393]
        tunnel: [_ _ w391] -> w377
        tunnel: [w383 _ _] -> w376
        frame "PolymorphicSubVI", "SubVI" {
          w390 = refnum<vi> refnum  # SubVI
          n116 = To More Specific Class(target class=w390, reference=w389, error in=w388) -> (specific class reference=w387:refnum<vi>, error out=w386:errorcluster)
          n117 = property class="SubVI"(reference=w387, error in=w386) -> ("Terms[]"=w385:refnum<vi>[])  [unwired: 2 out]
          n118 = call <userlib>:"Terminals - Filter invalid Terms.vi"("Terms[]"=w385) -> ("Terms[] out"=w384:refnum<vi>[])  [unwired: 10 in]
          n119 = call <userlib>:"Terminals - Filter Indicator Terms.vi"("Terms[]"=w384) -> ("Terms[] out"=w383:refnum<vi>[])  [unwired: 10 in]
        }
        frame Default {
        }
        frame "StringConstant" {
          w394 = refnum<vi> refnum  # StringConstant
          n120 = To More Specific Class(target class=w394, reference=w395, error in=w393) -> (specific class reference=w392:refnum<vi>)  [unwired: 1 out]
          n121 = Build Array(w392) -> (w391:refnum<vi>[])
        }
      }
    }
    n122 = Build Array (concatenate)(w366, w368) -> (w367:refnum<vi>[])
    n123 = Empty Array?(array=w367) -> (empty?=w369:bool)
  }
  n124 = call-poly <userlib>:"CSM-Helper API.vi"("error in (no error)"=w6, "CSM-Helper in"=w7) -> ("error out"=w14:errorcluster)  [unwired: 8 in, 1 out]
  n125 = flat-sequence {
    tunnel: w14 -> [_]
    frame #0 {
      n126 = call <userlib>:"CSM - Send Message and Wait for Reply.vi"("Target Module"="CSM", "State"="Macro: Exit") -> ()  [unwired: 7 in, 3 out]
    }
  }
  n127 = for {
    tunnel: w2 -> [w399] mode=indexing
    tunnel: [w398] -> w1 mode=indexing
    n128 = property class="StrCnst"(reference=w399) -> ("Text.Text"=w398:string)  [unwired: 1 in, 2 out]
  }
  "Array" <- w1
